vi "Fast IV Contour V2.vi"(8 "error in":errorcluster, 11 "Book number":i32=511) -> (0 "error out":errorcluster)   [LabVIEW 2021]
uses:
  <vilib>/Utility/file.llb/Write Delimited Spreadsheet (DBL).vi
panel:
  out "IV":cluster{dbl[], dbl[]}(graph)
  in  "Tab Control":enum32{"Set IV DAQ", "Set waveform", "Scan"}(tab)=enum."Scan"
  in  "rate":dbl=100000.0 format="%#_13g"
  in  "Trigger source":tag="/Dev1/PFI12"
  in  "samples per channel":i32=2000
  in  "Voltage Read":tag="Dev1/ai1, Dev1/ai2"
  in  "Voltage Scale factor":dbl=0.0001
  in  "Current Scale factor":dbl=1.0
  in  "Measurement  range V":dbl=10.0
  in  "V Amp V":dbl=0.8
  in  "Frequency Hz":dbl=50.0
  in  "Select Waveform device":string(combo)="Agilent 33250A"
  in  "Field step mT":dbl=0.1 format="%#_13g"
  in  "Average times":i32=20
  in  "Field Origin mT":dbl=-6.0 format="%#_13g"
  in  "Field Radius mT":dbl=12.0 format="%#_13g"
  in  "Ramp type":string(combo)="Range"
  in  "Magnet Device Select":string(combo)="Elsa Magnet"
  in  "Ramp up first T":bool=TRUE
  out "Current Field mT":dbl=6.0
  in  "Field Rate mT per sec":dbl=0.1 format="%#_13g"
  in  "Contour plot folder":path=path "C:/Users/gyue/Box Sync/Guang Yue/data/Contour plot"
  # "Scale * Vread=V"
  # "Scale * Vread=uA"
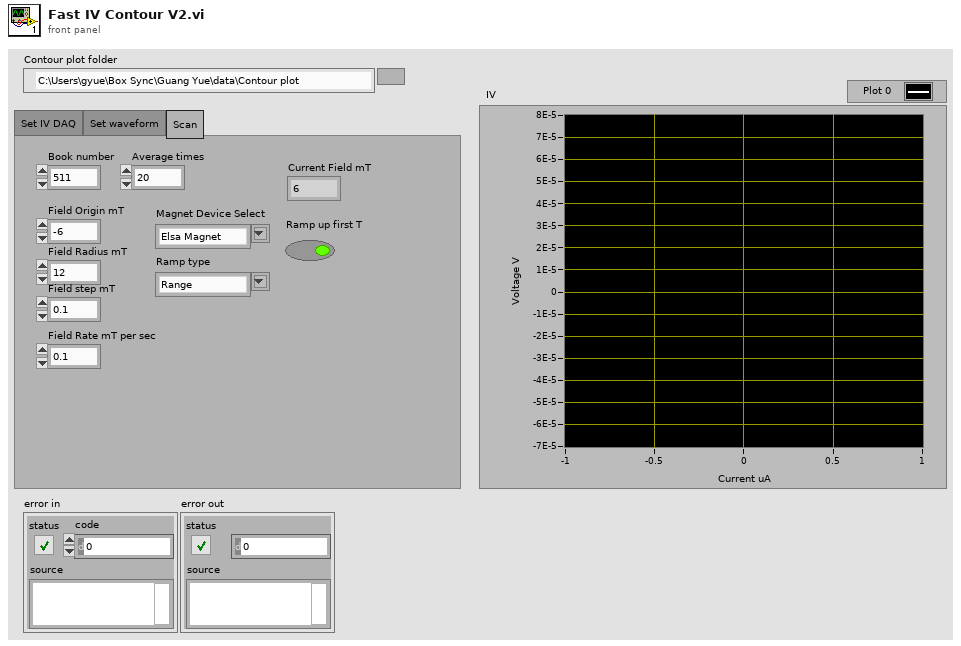
[diagram p1: front panel]
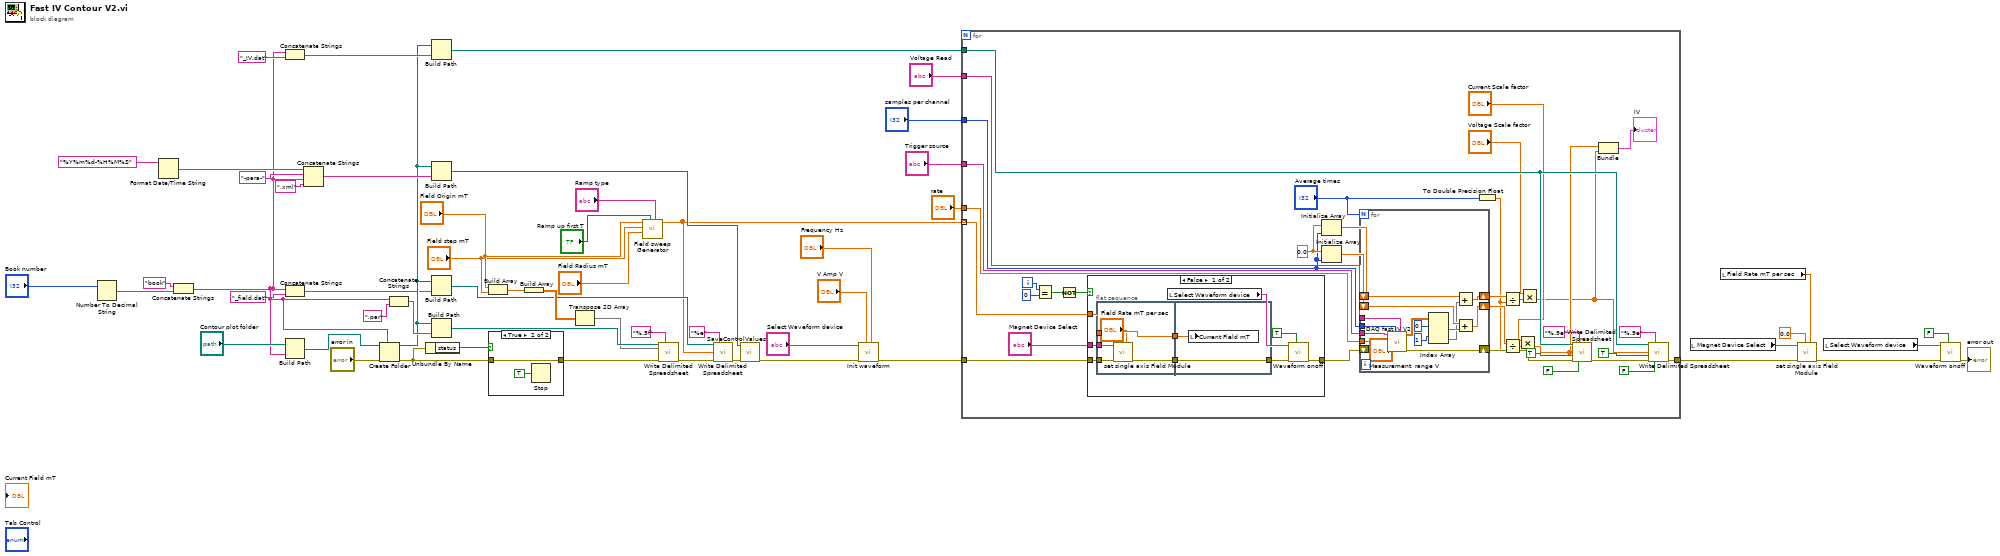
[diagram p0: block diagram]
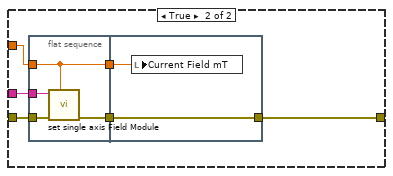
[diagram p3: hidden frame]
diagram:
  n1 = Number To Decimal String(number="Book number") -> (decimal integer string=w33:string)  [unwired: 1 in]
  n2 = Format Date/Time String(time format string (%c)="%Y%m%d-%H%M%S") -> (date/time string=w39:string)  [unwired: 2 in]
  n3 = Concatenate Strings("book" ("string"), w33) -> (w26:string)
  n4 = Concatenate Strings(w26, "_IV.dat" ("string")) -> (w46:string)
  n5 = Concatenate Strings(w26, "_field.dat" ("string")) -> (w27:string)
  n6 = Build Path(base path="Contour plot folder", name or relative path=w26) -> (appended path=w43:path)
  n7 = Concatenate Strings(w39, "-para-" ("string"), w26, ".xml" ("string")) -> (w54:string)
  n8 = Create Folder(prompt (Create Folder)=w26, path (use dialog)=w43, error in="error in") -> (created path=w28:path, error out=w41:errorcluster)  [unwired: 1 out]
  n9 = Concatenate Strings(w26, ".par" ("string")) -> (w50:string)
  n10 = Unbundle By Name(w41) -> ("status"=w42:bool)
  n11 = Build Path(base path=w28, name or relative path=w46) -> (appended path=w45:path)
  n12 = Build Path(base path=w28, name or relative path=w54) -> (appended path=w52:path)
  n13 = Build Path(base path=w28, name or relative path=w27) -> (appended path=w17:path)
  n14 = Build Path(base path=w28, name or relative path=w50) -> (appended path=w49:path)
  n15 = Build Array("Field Origin mT", "Field step mT") -> (w23:dbl[])
  n16 = case shown="True" w42 {
    tunnel: [w57 w59] -> w40
    tunnel: w41 -> [w57 w59]
    frame False {
    }
    frame True {
      n17 = Stop(stop? (T)=TRUE) -> ()
    }
  }
  n18 = Build Array(w23) -> (w22:dbl[][])
  n19 = Transpose 2D Array(2D array=w22) -> (transposed array=w19:dbl[][])
  n20 = call "Field sweep Generator.vi"("Ramp type"="Ramp type", "Ramp up first T"="Ramp up first T", "Field Radius"="Field Radius mT", "Field step"="Field step mT", "Field Origin"="Field Origin mT") -> ("output array"=w9:dbl[])  [unwired: 6 in]
  n21 = call-poly <vilib>:"Write Delimited Spreadsheet.vi"("file path (dialog if empty)"=w49, "format (%.3f)"="%.5f", "2D data"=w19, "error in (no error)"=w40) -> ("error out"=w16:errorcluster)  [unwired: 10 in, 1 out]
  n22 = call-poly <vilib>:"Write Delimited Spreadsheet.vi"("file path (dialog if empty)"=w17, "format (%.3f)"="%e", "1D data"=w9, "error in (no error)"=w16) -> ("error out"=w15:errorcluster)  [unwired: 10 in, 1 out]
  n23 = call "SaveControlValues.vi"("XML File Path"=w52, "error in (no error)"=w15) -> ("error out"=w14:errorcluster)  [unwired: 8 in]
  n24 = call "Init waveform.vi"("Frequency Hz"="Frequency Hz", "Vamp V"="V Amp V", "error in"=w14, "Select device"="Select Waveform device") -> ("error out"=w10:errorcluster)  [unwired: 7 in]
  n25 = for {
    tunnel: w45 -> [w68]
    tunnel: w10 -> [w91]
    tunnel: [w67] -> w8
    tunnel: "Voltage Read" -> [w88]
    tunnel: "samples per channel" -> [w76]
    tunnel: "Trigger source" -> [w87]
    tunnel: "rate" -> [w86]
    tunnel: w9 -> [w81] mode=indexing
    i -> [w82]
    w77 = 0.0 ("element")
    n26 = Equal?(x=w82, y=0) -> (x = y?=w92:bool)
    n27 = Not(x=w92) -> (.not. x?=w79:bool)
    n28 = case shown="False" w79 {
      tunnel: w91 -> [w120 w130]
      tunnel: [w112 w128] -> w90
      tunnel: w81 -> [w119 w129]
      tunnel: "Magnet Device Select" -> [w116 w131]
      frame False {
        n29 = flat-sequence {
          tunnel: w120 -> [w125]
          tunnel: w119 -> [w124]
          tunnel: [w124] -> w118
          tunnel: [w123] -> w117
          tunnel: w116 -> [w122]
          tunnel: w118 -> [w127]
          tunnel: [w126] -> w115
          tunnel: w117 -> [w126]
          frame #0 {
            n30 = call "set single axis Field Module.vi"("Field Rate mT per sec"="Field Rate mT per sec", "Field Target mT"=w124, "error in (no error)"=w125, "Device Select"=w122) -> ("error out"=w123:errorcluster)  [unwired: 7 in]
          }
          frame #1 {
            n31 = local write "Current Field mT"(w127) -> ()
          }
        }
        n32 = local read "Select Waveform device"() -> (w114:string)
        n33 = call "Waveform onoff.vi"("Enable Output  (T: Enable)"=TRUE, "error in"=w115, "Select device"=w114) -> ("error out"=w112:errorcluster)  [unwired: 8 in]
      }
      frame True {
        n34 = flat-sequence {
          tunnel: w130 -> [w137]
          tunnel: w129 -> [w136]
          tunnel: [w136] -> w133
          tunnel: [w135] -> w132
          tunnel: w131 -> [w134]
          tunnel: w133 -> [w139]
          tunnel: [w138] -> w128
          tunnel: w132 -> [w138]
          frame #0 {
            n35 = call "set single axis Field Module.vi"("Field Target mT"=w136, "error in (no error)"=w137, "Device Select"=w134) -> ("error out"=w135:errorcluster)  [unwired: 8 in]
          }
          frame #1 {
            n36 = local write "Current Field mT"(w139) -> ()
          }
        }
      }
    }
    n37 = Initialize Array(w77, w76) -> (w78:dbl[])
    n38 = Initialize Array(w77, w76) -> (w83:dbl[])
    n39 = for {
      N: "Average times" -> [_]
      tunnel: w88 -> [w109]
      tunnel: w76 -> [w108]
      tunnel: w87 -> [w107]
      tunnel: w86 -> [w106]
      shift-right: [w110] -> w89
      shift-left: w90 -> [w111]
      shift-right: [w105] -> w85
      shift-left: w83 -> [w104]
      shift-right: [w97] -> w75
      shift-left: w78 -> [w103]
      n40 = call "DAQ fast IV V2.vi"("physical channels I and V"=w109, "Measurement  range V"="Measurement  range V", "samples per channel"=w108, "error in"=w111, "rate"=w106, "Trigger source"=w107) -> ("error out"=w110:errorcluster, "Output"=w102:dbl[][])  [unwired: 4 in]
      n41 = Index Array(array=w102, index (row) #1=0 ("index (row)"), index (row) #2=1 ("index (row)")) -> (element #1=w100:dbl[], element #2=w98:dbl[])  [unwired: 2 in]
      n42 = Add(x=w103, y=w98) -> (x+y=w97:dbl[])
      n43 = Add(x=w104, y=w100) -> (x+y=w105:dbl[])
    }
    n44 = To Double Precision Float(number="Average times") -> (double precision float=w74:dbl)
    n45 = Divide(x=w75, y=w74) -> (x/y=w65:dbl[])
    n46 = Divide(x=w85, y=w74) -> (x/y=w66:dbl[])
    n47 = Multiply(x="Current Scale factor", y=w66) -> (x*y=w62:dbl[])
    n48 = Multiply(x="Voltage Scale factor", y=w65) -> (x*y=w61:dbl[])
    n49 = call-poly <vilib>:"Write Delimited Spreadsheet.vi"("file path (dialog if empty)"=w68, "format (%.3f)"="%.9e", "1D data"=w62, "append to file? (new file:F)"=TRUE ("append to file? (F)"), "error in (no error)"=w89, "transpose? (no:F)"=FALSE) -> ("error out"=w69:errorcluster)  [unwired: 8 in, 1 out]
    n50 = Bundle(w62, w61) -> (→"IV":cluster{dbl[], dbl[]})  [unwired: 1 in]
    n51 = call-poly <vilib>:"Write Delimited Spreadsheet.vi"("file path (dialog if empty)"=w68, "format (%.3f)"="%.9e", "1D data"=w61, "append to file? (new file:F)"=TRUE ("append to file? (F)"), "error in (no error)"=w69, "transpose? (no:F)"=FALSE) -> ("error out"=w67:errorcluster)  [unwired: 8 in, 1 out]
  }
  n52 = local read "Magnet Device Select"() -> (w7:string)
  n53 = local read "Field Rate mT per sec"() -> (w1:dbl)
  n54 = call "set single axis Field Module.vi"("Field Rate mT per sec"=w1, "Field Target mT"=0.0, "error in (no error)"=w8, "Device Select"=w7) -> ("error out"=w5:errorcluster)  [unwired: 7 in]
  n55 = local read "Select Waveform device"() -> (w4:string)
  n56 = call "Waveform onoff.vi"("Enable Output  (T: Enable)"=FALSE, "error in"=w5, "Select device"=w4) -> ("error out"=→"error out":errorcluster)  [unwired: 8 in]
